vi "Pack for gRPC.vi"(8 "error in":errorcluster, 9 "configuration / results":enum16{"Configuration", "Results"}(ring), 10 "data value":variant, 11 "measurement customizations in":refnum<class "Measurement Plugin.lvclass">) -> (0 "error out":errorcluster, 2 "any":T1, 3 "measurement customizations out":refnum<class "Measurement Plugin.lvclass">)   [LabVIEW 2021, in "Crosstalk_Audio DAC.lvlib" / "Measurement Plugin.lvclass"]
uses:
  Measurement Plugin.lvclass
  <vilib>/gRPC/LabVIEW gRPC Library/Shared/Any.ctl
  C:/Program Files/National Instruments/LabVIEW 2021/vi.lib/MeasurementLink/MeasurementLink Measurement Server/Measurement Plugin Service/Measurement Plugin Service.lvclass
  Measurement Configuration.ctl
  Measurement Results.ctl
  2eca732d-dbaa-43bf-a7dd-ede2da65bc1b.vi
  a6012965-5700-4384-8228-972e71b6560c.vi
  <vilib>/gRPC/LabVIEW gRPC Library/Server API/Translate Protobuf Error.vi
  <vilib>/AdvancedString/1D String Array to Delimited String.vi
  <vilib>/gRPC/LabVIEW gRPC Library/Server API/Server/Get Server DLL Path.vi
  Measurement Plugin.lvclass/Measurement Plugin.ctl
  Crosstalk_Audio DAC.lvlib
  <vilib>/MeasurementLink/MeasurementLink Measurement Server/Measurement Plugin Service/Measurement Plugin Service.lvclass
  <vilib>/gRPC/LabVIEW gRPC Library/grpc-lvsupport-release.lvlib
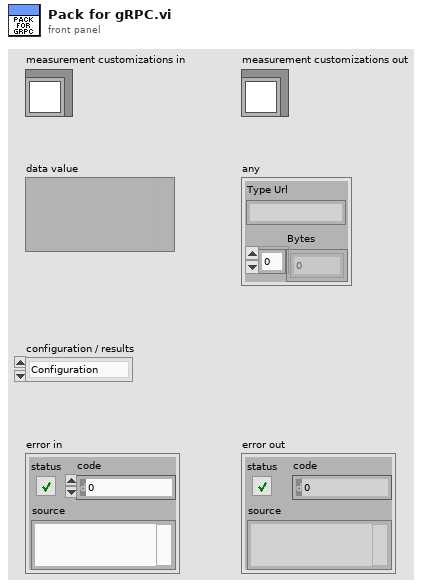
[diagram p1: front panel]
types:
  T1 = typedef "grpc-lvsupport-release.lvlib/Any.ctl" = cluster{"Type Url":string, "Bytes":u8[]}
  T2 = typedef "grpc-lvsupport-release.lvlib/grpcId.ctl" = u64
  T3 = typedef "Crosstalk_Audio DAC.lvlib/Measurement Configuration.ctl" = cluster{"Frequency (Hz)":dbl, "Protocol file":string, "Digital audio channel":string, "Master clock channel":string, "Output level":dbl, "Output level units":string, "Output range (Vpk-pk)":dbl, "Victim channel resource":string, "Interferrer channel resource":string, "Sample rate (Hz)":dbl, "Min measurement cycles":u32, "Min measurement time (s)":dbl, "Min settling cycles":u32, "Min settling time (s)":dbl, "Highpass filter":string, "Lowpass filter":string, "Weighting filter":string, "Band start (Hz)":dbl, "Band stop (Hz)":dbl, "Interferrer channel":string}
  T4 = typedef "Crosstalk_Audio DAC.lvlib/Measurement Results.ctl" = cluster{"Channel names":string[], "Time domain":dbl[], "Frequency domain":dbl[], "dt":dbl, "f0":dbl, "df":dbl, "Frequency":dbl[], "Crosstalk":dbl[]}
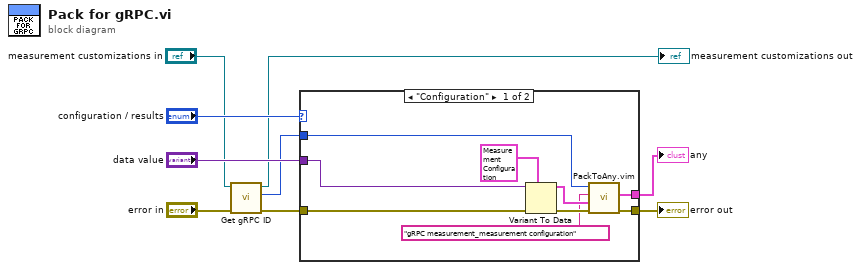
[diagram p0: block diagram]
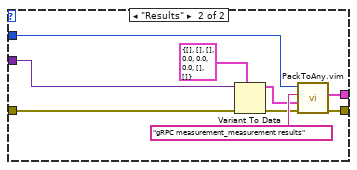
[diagram p2: hidden frame]
diagram:
  n1 = call <vilib>:"Get gRPC ID.vi"("error in"="error in", "measurement plugin service in"="measurement customizations in") -> ("error out"=w4:errorcluster, "gRPC ID"=w1:T2, "measurement plugin service out"=→"measurement customizations out":refnum<class "Measurement Plugin.lvclass">)  [unwired: 7 in]
  n2 = case shown="\"Configuration\"" "configuration / results" {
    tunnel: w4 -> [w18 w27]
    tunnel: "data value" -> [w17 w26]
    tunnel: w1 -> [w14 w22]
    tunnel: [w16 w24] -> w8
    tunnel: [w15 w23] -> w7
    frame "Configuration" {
      n3 = Variant To Data(error in=w18, type=T3 {"Frequency (Hz)"=1000.0, "Protocol file"="", "Digital audio channel"="", "Master clock channel"="", "Output level"=0.0, "Output level units"="dBFS", "Output range (Vpk-pk)"=5.74, "Victim channel resource"="", "Interferrer channel resource"="", "Sample rate (Hz)"=51200.0, "Min measurement cycles"=0, "Min measurement time (s)"=0.1, "Min settling cycles"=0, "Min settling time (s)"=0.1, "Highpass filter"="AC", "Lowpass filter"="AES17_20kHz", "Weighting filter"="A-weighting", "Band start (Hz)"=20.0, "Band stop (Hz)"=20000.0, "Interferrer channel"=""} ("measurement configuration"), Variant=w17) -> (data=w13:T3, error out=w12:errorcluster)
      n4 = call "PackToAny.vim"("error in"=w12, "Data To Pack"=w13, "Message Type"="gRPC measurement_measurement configuration", "gRPCid in"=w14) -> ("error out"=w16:errorcluster, "Any"=w15:T1)  [unwired: 5 in, 1 out]
    }
    frame "Results" {
      n5 = Variant To Data(error in=w27, type=T4 {"Channel names"=[], "Time domain"=[], "Frequency domain"=[], "dt"=0.0, "f0"=0.0, "df"=0.0, "Frequency"=[], "Crosstalk"=[]} ("Measurement Results"), Variant=w26) -> (data=w20:T4, error out=w19:errorcluster)
      n6 = call "PackToAny.vim"("error in"=w19, "Data To Pack"=w20, "Message Type"="gRPC measurement_measurement results", "gRPCid in"=w22) -> ("error out"=w24:errorcluster, "Any"=w23:T1)  [unwired: 5 in, 1 out]
    }
  }
  "error out" <- w8
  "any" <- w7
